vi "Get CoPilot Queue Ref.vi"(8 "Error In":errorcluster) -> (0 "Error Out":errorcluster, 3 "queue out":refnum<queue>)   [LabVIEW 2014]
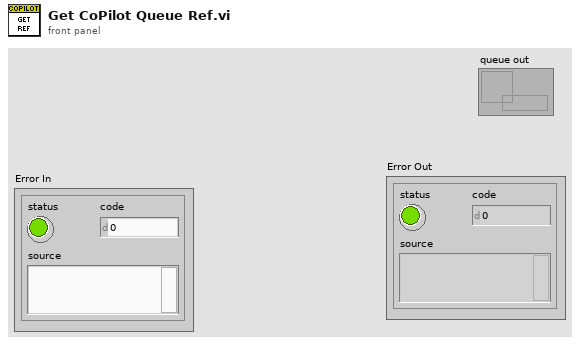
[diagram p1: front panel]
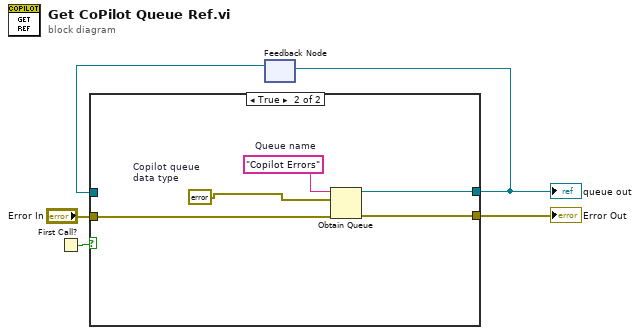
[diagram p0: block diagram]
diagram:
  n1 = First Call?() -> (First Call?: T/F=w5:bool)
  n2 = feedback #1() -> (w3:refnum<queue>)  [unwired: 1 in]
  n3 = case shown="True" w5 {
    tunnel: [w6 w10] -> w2
    tunnel: [w7 w9] -> w4
    tunnel: w3 -> [w7 _]
    tunnel: "Error In" -> [w6 w8]
    frame False {
    }
    frame True {
      w11 = errorcluster {"status"=FALSE, "code"=0, "source"=""}  # Copilot queue  data type
      w12 = "Copilot Errors"  # Queue name
      n4 = Obtain Queue(name (unnamed)=w12, element data type=w11, error in (no error)=w8) -> (queue out=w9:refnum<queue>, error out=w10:errorcluster)  [unwired: 2 in, 1 out]
    }
  }
  "Error Out" <- w2
  "queue out" <- w4
  n5 = feedback-in #1(w4) -> ()
